vi "oax_GS Order Magnitude and Phase.vi"(0 "scaled signals [EU]":waveform(dbl)[](array[waveform]), 1 "X axis selection":u16, 2 "magnitude view":enum16{"no change", "rms", "peak", "peak-peak"}(ring), 3 "bandwidth [order]":dbl, 5 "speed profile":T2 {"speed [RPM]" format="%.2f"; "time [s]" format="%.2f"}, 7 "orders to track":dbl[](array[numeric]), 9 "select channel":u16, 11 "error in (no error)":errorcluster, 12 "max order to analyze":dbl, 13 "pulse/rev":i32, 14 "view":T4) -> (4 "magnitude":T3(array[cluster]), 6 "phase":cluster{"time/rev/rpm":dbl[], "phase":dbl[]}[](array[cluster]), 8 "unit label":T1, 15 "error out":errorcluster)   [LabVIEW 2017]
uses:
  <vilib>/addons/Sound and Vibration/Order Analysis/Tach Process/SubVIs/speed profile.ctl
  <vilib>/addons/_NISVFA/_Spectrum Processing/SVFA Unit Conversion (XY) (N Ch).vi
  <vilib>/addons/Sound and Vibration/Order Analysis/Resample Order Tracking/OAT Order Magnitude and Phase (Even Angle Signal, N Channels).vi
  <vilib>/addons/Sound and Vibration/Order Analysis/Resample Order Tracking/OAT Convert to Even Angle Signal (N Channels).vi
  <vilib>/addons/Sound and Vibration/Order Analysis/Resample Order Tracking/SoundVib_OrderTracking.lvlib
  <vilib>/addons/Sound and Vibration/Order Analysis/Tach Process/SoundVib_TachProcess.lvlib
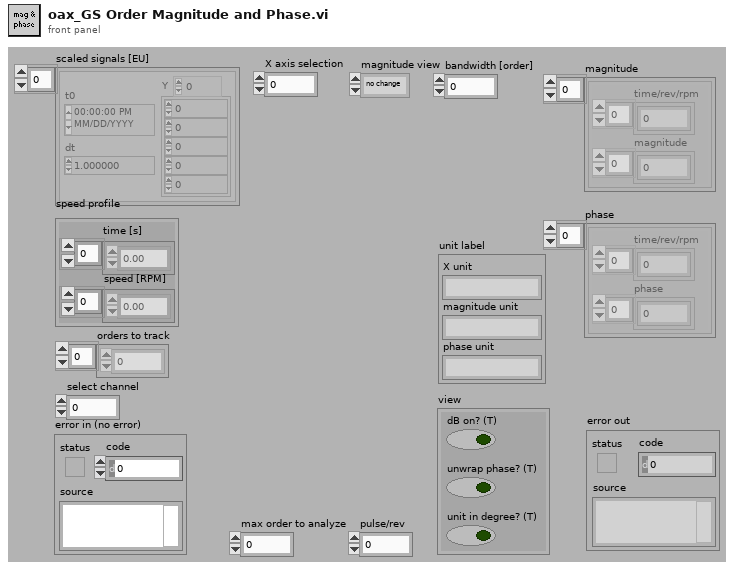
[diagram p1: front panel]
types:
  T1 = cluster{"X unit":string, "magnitude unit":string, "phase unit":string}
  T2 = typedef "SoundVib_TachProcess.lvlib/speed profile.ctl" = cluster{"time [s]":dbl[], "speed [RPM]":dbl[]}
  T3 = cluster{"time/rev/rpm":dbl[], "magnitude":dbl[]}[]
  T4 = cluster{"dB on? (T)":bool, "unwrap phase? (T)":bool, "unit in degree? (T)":bool}
  T5 = cluster{"linear/dB":enum16{"no change", "linear", "dB"}, "dB reference (0: no change)":dbl, "power/magnitude":enum16{"no change", "power", "magnitude"}, "view":enum16{"no change", "rms", "peak", "peak-peak"}}
  T6 = typedef "svc_Resampled Channel Info.ctl" = cluster{"channel name":string, "description":string, " channel info":T7}
  T7 = typedef "svc_Channel Info.ctl" = cluster{"sensor sensitivity":dbl, "engineering units":T8, "dB reference":dbl, "custom label":string, "weighting filter":T9, "pregain":dbl}
  T8 = typedef "svc_Engineering Units Text Ring.ctl" = u16
  T9 = typedef "svc_Weighting Filter Text Ring.ctl" = u16
  T10 = typedef "OAT Position Info.ctl" = cluster{"positions [s]":dbl[], "samples/rev":dbl}
  T11 = cluster{"x unit":string, "magnitude unit":string, "phase unit":string}[]
  T12 = cluster{"time/rev/rpm":dbl[], "magnitude":dbl[]}[][]
  T13 = typedef "svc_Spectrum Info.ctl" = cluster{"channel name":string, "description":string, "x-axis units":T14, "spectral info":cluster{"spectrum type":T15, "linear/dB":enum16{"linear", "dB"}, "window":u16, "window size":i32, "FFT size":i32}, "engineering units":T8, "custom label":string, "dB reference [EU]":dbl, "peak units":enum16{"rms", "peak", "peak-peak"}, "weighting filter":T9, "spectral density?":bool, "unit label":string, "spectrum skewed?":bool, "complimentary spectrum units":T16}
  T14 = typedef "svc_X-Axis Units.ctl" = u16
  T15 = typedef "svc_Spectrum Type.ctl" = enum16{"FFT Spectrum [complex]", "Amplitude [Magnitude]", "Power [Magnitude^2]", "Cross Spectrum [complex]", "Frequency Response [Complex]"}
  T16 = typedef "svc_Complimentary Spectrum Units.ctl" = enum16{"none", "radians", "degrees", "cycles", "imaginary"}
  T17 = cluster{"x unit":string, "magnitude unit":string, "phase unit":string}
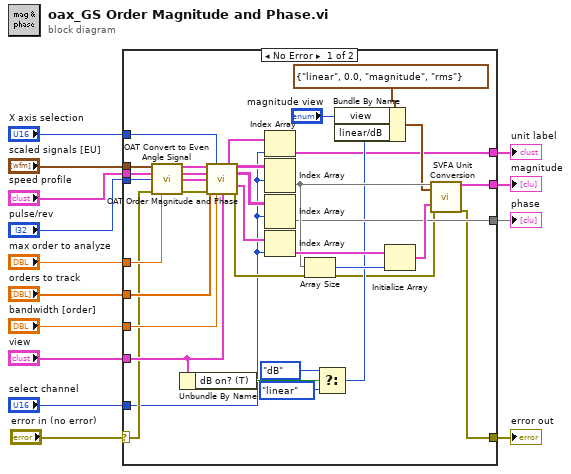
[diagram p0: block diagram]
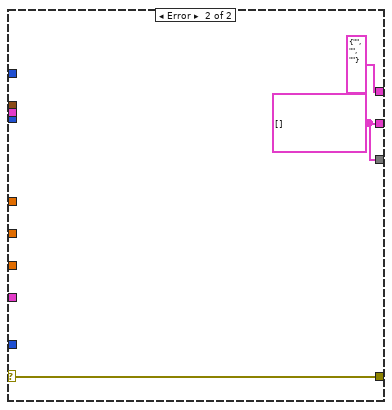
[diagram p2: hidden frame]
diagram:
  n1 = case shown="No Error" "error in (no error)" {
    selector: "error in (no error)" -> [w20 w51]
    tunnel: "pulse/rev" -> [w48 _]
    tunnel: "max order to analyze" -> [w47 _]
    tunnel: "scaled signals [EU]" -> [w46 _]
    tunnel: "orders to track" -> [w45 _]
    tunnel: "select channel" -> [w16 _]
    tunnel: [w34 w50] -> w9
    tunnel: [w33 w50] -> w8
    tunnel: "X axis selection" -> [w30 _]
    tunnel: "bandwidth [order]" -> [w29 _]
    tunnel: "speed profile" -> [w28 _]
    tunnel: "view" -> [w26 _]
    tunnel: [w19 w51] -> w2
    tunnel: [w15 T1 {"X unit"="", "magnitude unit"="", "phase unit"=""} ("unit labels")] -> w1
    frame No Error {
      n2 = call-poly <vilib>:"OAT Convert to Even Angle Signal.vi"("scaled signals [EU]"=w46, "speed profile"=w28, "pulse/revolution (1)"=w48, "error in (no error)"=w20, "max order (auto)"=w47) -> ("even-angle signals"=w43:cluster{"r0":dbl, "dr":dbl, "Y":dbl[]}[], "even-angle channel info"=w44:T6[], "even-angle position info"=w27:T10, "error out"=w21:errorcluster)  [unwired: 6 in, 1 out]
      n3 = Unbundle By Name(w26) -> ("dB on? (T)"=w25:bool)
      n4 = call-poly <vilib>:"OAT Order Magnitude and Phase.vi"("even-angle signals"=w43, "x-axis selection"=w30, "even-angle channel info"=w44, "even-angle position info"=w27, "orders to compute (1.0)"=w45, "error in (no error)"=w21, "bandwidth [order]"=w29, "view"=w26) -> ("unit labels"=w17:T11, "magnitudes [RMS]"=w31:T12, "phases [phase lag]"=w32:cluster{"time/rev/rpm":dbl[], "phase":dbl[]}[][], "magnitudes info"=w35:T13[], "error out"=w18:errorcluster)  [unwired: 2 in, 1 out]
      n5 = Index Array(array=w17, index=w16) -> (element=w15:T17)
      n6 = Index Array(array=w31, index (row)=w16) -> (element=w40:T3)  [unwired: 1 in]
      n7 = Index Array(array=w32, index (row)=w16) -> (element=w33:cluster{"time/rev/rpm":dbl[], "phase":dbl[]}[])  [unwired: 1 in]
      n8 = Index Array(array=w35, index=w16) -> (element=w42:T13)
      n9 = Array Size(array=w40) -> (size(s)=w41:i32)
      n10 = Select(t=enum16{"no change", "linear", "dB"}."dB" ("linear/dB"), s=w25, f=enum16{"no change", "linear", "dB"}."linear" ("linear/dB")) -> (s? t:f=w22:enum16{"no change", "linear", "dB"})
      n11 = Bundle By Name(cluster=T5 {"linear/dB"=enum."linear", "dB reference (0: no change)"=0.0, "power/magnitude"=enum."magnitude", "view"=enum."rms"} ("desired scaling"), "view"="magnitude view", "linear/dB"=w22) -> (w38:T5)
      n12 = Initialize Array(w42, w41) -> (w39:T13[])
      n13 = call-poly <vilib>:"SVFA Unit Conversion.vi"("magnitudes"=w40, "desired scaling"=w38, "magnitudes info in"=w39, "error in (no error)"=w18) -> ("converted magnitudes"=w34:T3, "error out"=w19:errorcluster)  [unwired: 12 in, 2 out]
    }
    frame Error {
      w50 = T3 [] ("converted magnitudes")
    }
  }
  "magnitude" <- w9
  "phase" <- w8
  "error out" <- w2
  "unit label" <- w1
